vi "LJM logger get error device open params.vi"() -> (0 "Serial Number":i32, 1 "Connection Type":string, 2 "Device Type":string)   [LabVIEW 2026]
panel:
  # "This VI provides consistent device open\nparameter error values if a connection\ncould not be established."
  # "Be sure to change LJM logger open constants to string.vi and LJM logger open with invalid device filter.vi if you change this VI."
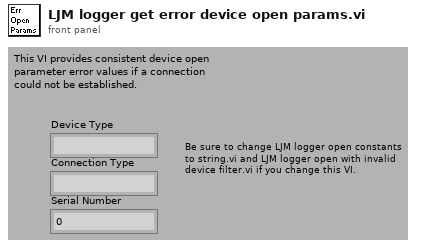
[diagram p1: front panel]
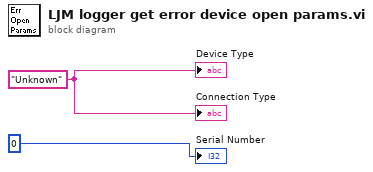
[diagram p0: block diagram]
diagram:
  w2 = "Unknown" ("DevTypeString")
  "Serial Number" <- 0 ("SerialNumber")
  "Device Type" <- w2
  "Connection Type" <- w2
